vi "send data FIX.vi"() -> ()   [LabVIEW 2016]
uses:
  <vilib>/Instr/_visa.llb/Select Event Type.ctl
  <vilib>/Utility/error.llb/DialogType.ctl
  <vilib>/Instr/_visa.llb/VISA Configure Serial Port (Instr).vi
  <vilib>/httpClient/LabVIEWHTTPClient.lvlib
  <vilib>/gmath/NI_Gmath.lvlib
panel:
  out "headers":string
  out "mean value":dbl
  out "error out":errorcluster
  out "body":string
  out "Current queue":dbl[](array[numeric])
  out "Last 15 values":dbl[](array[numeric])
  out "Internet OK":bool
  out "read buffer":string
  out "Waveform Chart":dbl(graph)
  out "recv bytes":u32
  in  "VISA resource name":refnum<visa-resource-name>
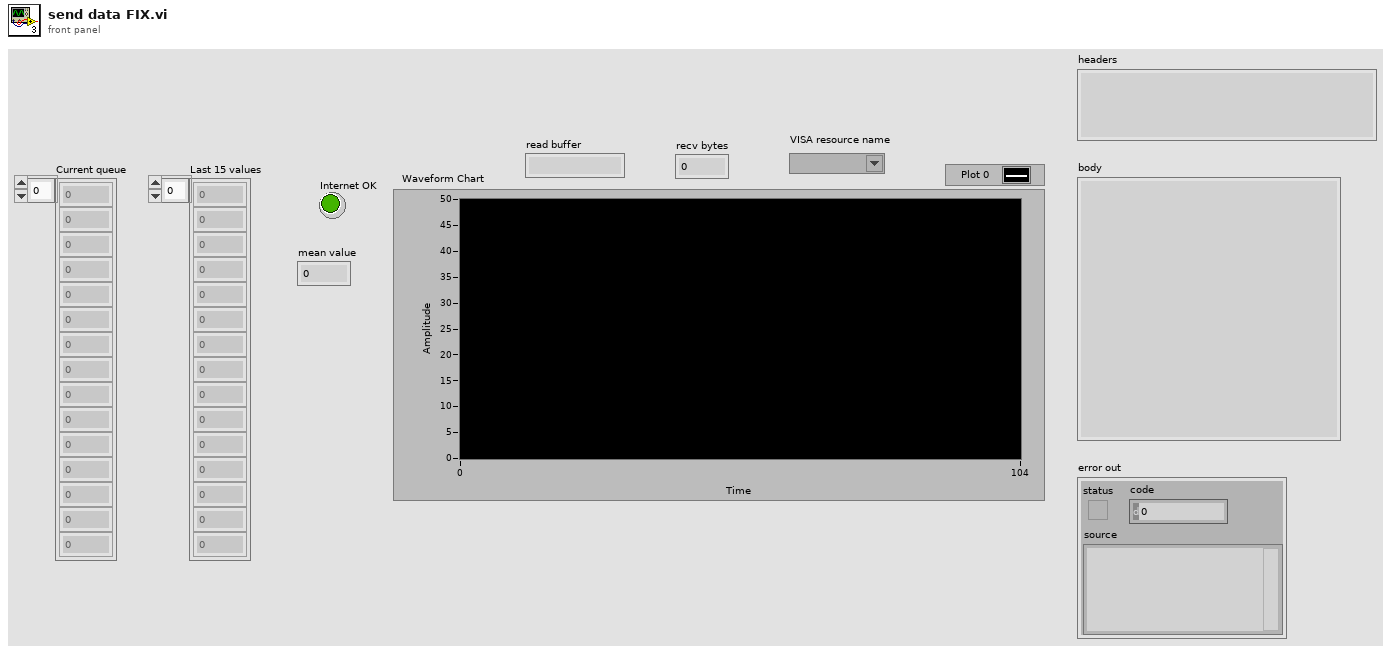
[diagram p1: front panel]
types:
  T1 = typedef "Select Event Type.ctl" = u32
  T2 = typedef "DialogType.ctl" = u16
  T3 = typedef "LabVIEWHTTPClient.lvlib/ClientHandle.ctl" = refnum<k1>
  T4 = enum16{"arithmetic", "geometric", "harmonic", "trimmed", "median"}
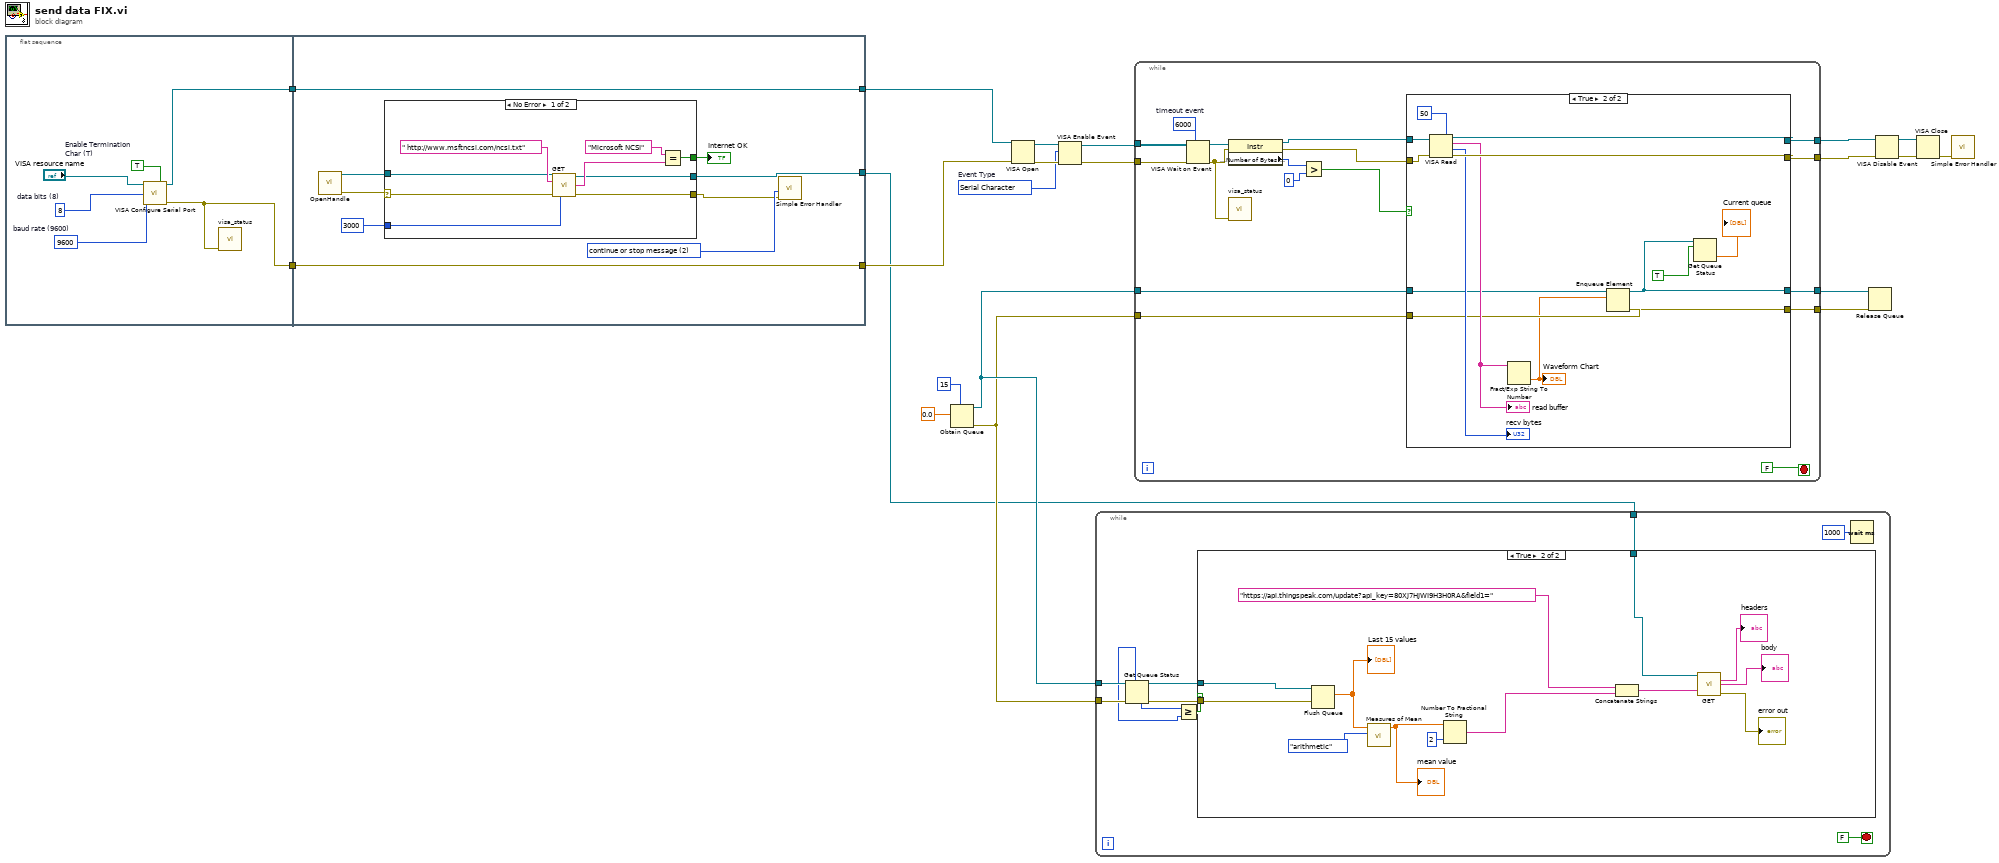
[diagram p0: block diagram]
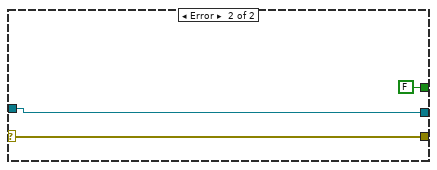
[diagram p4: hidden frame]
diagram:
  w12 = T1 1073684533 items=["Service Request"=1073684491, "Trigger"=3221168138, "Clear"=1073684493, "VXI Signal"=1073684512, "VXI/VME Interrupt"=3221168161, "VXI/VME Sysfail"=1073684509, "VXI/VME Sysreset"=1073684510, "GPIB CIC"=1073684498, "GPIB Talk"=1073684499, "GPIB Listen"=1073684500, "PXI Interrupt"=1073684514, "Serial Break"=1073684515, "Serial TermChar"=1073684516, "Serial CTS"=1073684521, "Serial DSR"=1073684522, "Serial DCD"=1073684524, "Serial RI"=1073684526, "Serial Character"=1073684533, "USB Interrupt"=1073684535, "All Enabled"=1073709055]  # Event Type
  n1 = flat-sequence {
    tunnel: [w23] -> w11
    tunnel: [w22] -> w8
    tunnel: w11 -> [w36]
    tunnel: [w36] -> w10
    tunnel: [w35] -> w9
    tunnel: w8 -> [w35]
    tunnel: [w28] -> w1
    frame #0 {
      w24 = u16 8  # data bits (8)
      w25 = TRUE  # Enable Termination Char (T)
      w26 = u32 9600  # baud rate (9600)
      n2 = call-poly "VISA Configure Serial Port"("VISA resource name"="VISA resource name", "Enable Termination\nChar (T)"=w25, "baud rate (9600)"=w26, "data bits (8)"=w24) -> ("VISA resource name out"=w22:refnum<visa-resource-name>, "error out"=w23:errorcluster)  [unwired: 10 in]
      n3 = call "visa_status.vi"("error in (no error)"=w23) -> ()  [unwired: 11 in]
    }
    frame #1 {
      w30 = T2 2 items=["no dialog", "OK message", "continue or stop message", "OK message + warnings", "continue/stop + warnings"] ("type of dialog (OK msg:1)")
      n4 = call <vilib>:"OpenHandle.vi"() -> ("client handle out"=w31:T3, "error out"=w32:errorcluster)  [unwired: 14 in]
      n5 = case shown="No Error" w32 {
        selector: w32 -> [w40 w47]
        tunnel: [w42 FALSE] -> w34
        tunnel: [w41 w47] -> w29
        tunnel: 3000 ("timeout (ms)") -> [w39 _]
        tunnel: w31 -> [w38 w46]
        tunnel: [w37 w46] -> w28
        frame No Error {
          n6 = call <vilib>:"GET.vi"("client handle"=w38, "url"=" http://www.msftncsi.com/ncsi.txt" ("address"), "error in (no error)"=w40, "timeout (10000)"=w39) -> ("client handle out"=w37:T3, "body"=w43:string, "error out"=w41:errorcluster)  [unwired: 8 in, 1 out]
          n7 = Equal?(x="Microsoft NCSI", y=w43) -> (x = y?=w42:bool)
        }
        frame Error {
        }
      }
      "Internet OK" <- w34
      n8 = call <vilib>:"Simple Error Handler.vi"("type of dialog (OK msg:1)"=w30, "error in (no error)"=w29) -> ()  [unwired: 3 in, 5 out]
    }
  }
  n9 = Obtain Queue(max queue size (-1, unlimited)=15, element data type=0.0) -> (queue out=w5:refnum<queue>, error out=w4:errorcluster)  [unwired: 3 in, 1 out]
  n10 = VISA Open(error in (no error)=w10, VISA resource name=w9) -> (VISA resource name=w21:refnum<visa-resource-name>, error out=w20:errorcluster)  [unwired: 3 in]
  n11 = VISA Enable Event(8:w20, 10:w12, 11:w21) -> (0:w18:errorcluster, 3:w19:refnum<visa-resource-name>)  [unwired: 1 in]
  n12 = while {
    tunnel: w5 -> [w58]
    tunnel: w4 -> [w57]
    tunnel: w1 -> [w49]
    stop <- FALSE stop-if-true
    n13 = Get Queue Status(queue=w58, error in (no error)=w57) -> (queue out=w54:refnum<queue>, max queue size=w50:i32, error out=w53:errorcluster, # elements in queue=w55:i32)  [unwired: 1 in, 4 out]
    n14 = Greater Or Equal?(x=w55, y=w50) -> (x >= y?=w56:bool)
    n15 = case shown="True" w56 {
      tunnel: w54 -> [_ w71]
      tunnel: w53 -> [_ w70]
      tunnel: w49 -> [_ w64]
      frame False {
      }
      frame True {
        n16 = Flush Queue(queue=w71, error in (no error)=w70) -> (remaining elements=w60:dbl[])  [unwired: 2 out]
        "Last 15 values" <- w60
        n17 = call <vilib>:"Measures of Mean.vi"("type"=T4."arithmetic", "x array"=w60) -> ("mean value"=w68:dbl)  [unwired: 8 in, 1 out]
        "mean value" <- w68
        n18 = Number To Fractional String(number=w68, precision (6)=i16 2) -> (F-format string=w66:string)  [unwired: 2 in]
        n19 = Concatenate Strings("https://api.thingspeak.com/update?api_key=80XJ7HJWI9H3H0RA&field1=" ("string"), w66) -> (w65:string)
        n20 = call <vilib>:"GET.vi"("client handle"=w64, "url"=w65) -> ("headers"=→"headers":string, "body"=→"body":string, "error out"=→"error out":errorcluster)  [unwired: 10 in, 1 out]
      }
    }
    n21 = Wait (ms)(milliseconds to wait=u32 1000) -> ()  [unwired: 1 out]
  }
  n22 = while {
    tunnel: w19 -> [w88]
    tunnel: w18 -> [w77]
    tunnel: [w87] -> w17
    tunnel: [w86] -> w16
    tunnel: w5 -> [w75]
    tunnel: w4 -> [w74]
    tunnel: [w73] -> w3
    tunnel: [w72] -> w2
    stop <- FALSE stop-if-true
    w79 = u32 6000  # timeout event
    n23 = VISA Wait on Event(7:w79, 8:w77, 11:w88) -> (0:w76:errorcluster, 3:w85:refnum<visa-resource-name>)  [unwired: 2 in, 2 out]
    n24 = call "visa_status.vi"("error in (no error)"=w76) -> ()  [unwired: 11 in]
    n25 = property class="Instr"(reference=w85, error in=w76) -> (reference out=w84:refnum<visa-resource-name>, error out=w80:errorcluster, "Serial Settings:Number of Bytes at Serial Port"=w83:u32)
    n26 = Greater?(x=w83, y=u32 0) -> (0:w81:bool)
    n27 = case shown="True" w81 {
      tunnel: [w92 w106] -> w87
      tunnel: [w91 w105] -> w86
      tunnel: w84 -> [w92 w101]
      tunnel: w80 -> [w91 w100]
      tunnel: w75 -> [w90 w99]
      tunnel: w74 -> [w89 w98]
      tunnel: [w90 w96] -> w72
      tunnel: [w89 w97] -> w73
      frame False {
      }
      frame True {
        n28 = VISA Read(VISA resource name=w101, byte count=u32 50, error in (no error)=w100) -> (VISA resource name out=w106:refnum<visa-resource-name>, read buffer=w102:string, return count=→"recv bytes":u32, error out=w105:errorcluster)
        "read buffer" <- w102
        n29 = Fract/Exp String To Number(string=w102) -> (number=w93:dbl)  [unwired: 3 in, 1 out]
        "Waveform Chart" <- w93
        n30 = Enqueue Element(queue=w99, element=w93, error in (no error)=w98) -> (queue out=w96:refnum<queue>, error out=w97:errorcluster)  [unwired: 1 in, 1 out]
        n31 = Get Queue Status(queue=w96, return elements? (F)=TRUE) -> (elements=→"Current queue":dbl[])  [unwired: 1 in, 7 out]
      }
    }
  }
  n32 = Release Queue(queue=w2, error in (no error)=w3) -> ()  [unwired: 1 in, 3 out]
  n33 = VISA Disable Event(8:w16, 11:w17) -> (0:w15:errorcluster, 3:w14:refnum<visa-resource-name>)  [unwired: 2 in]
  n34 = VISA Close(VISA resource name=w14, error in (no error)=w15) -> (error out=w13:errorcluster)
  n35 = call <vilib>:"Simple Error Handler.vi"("error in (no error)"=w13) -> ()  [unwired: 4 in, 5 out]
